vi "13-2 시리얼통신.vi"() -> ()   [LabVIEW 2014]
uses:
  <vilib>/Instr/_visa.llb/VISA Configure Serial Port (Instr).vi
panel:
  in  "설정":bool
  in  "TH500 통신":bool
  in  "정지":bool
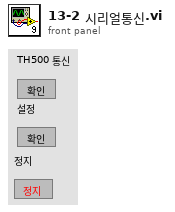
[diagram p1: front panel]
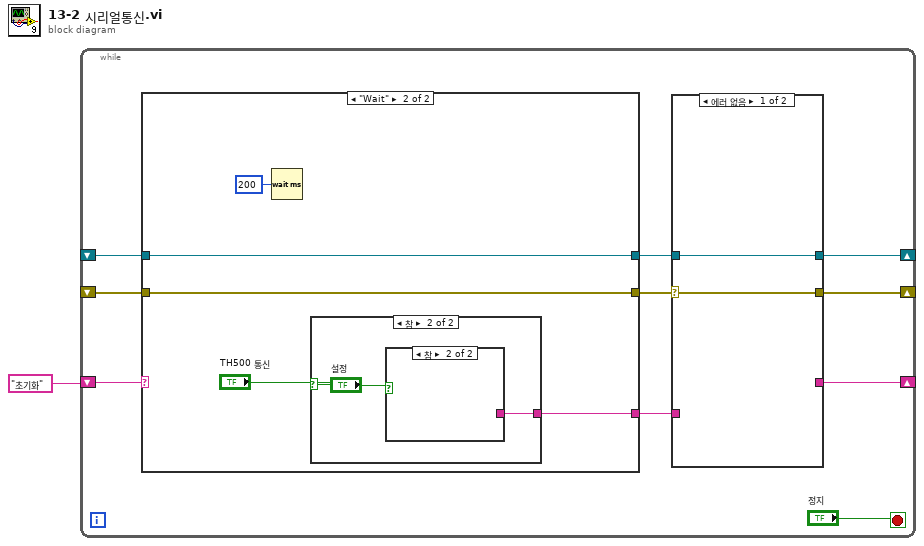
[diagram p0: block diagram]
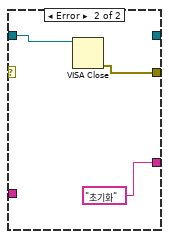
[diagram p2: hidden frame]
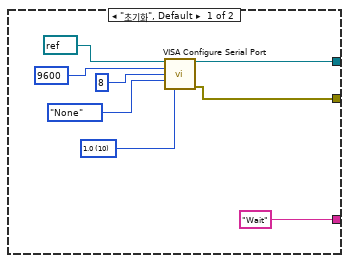
[diagram p3: hidden frame]
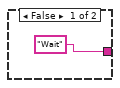
[diagram p4: hidden frame]
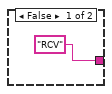
[diagram p5: hidden frame]
diagram:
  n1 = while {
    shift-right: [w6] -> _
    shift-left: _ -> [w2]
    shift-right: [w5] -> _
    shift-left: _ -> [w3]
    shift-right: [w4] -> _
    shift-left: "초기화" -> [w11]
    stop <- "정지" stop-if-true
    n2 = case shown="\"Wait\"" w11 {
      tunnel: ["Wait" w26] -> w9
      tunnel: [w18 w29] -> w8
      tunnel: [w17 w28] -> w7
      tunnel: w3 -> [_ w29]
      tunnel: w2 -> [_ w28]
      frame "초기화", Default {
        w20 = u16 10 items=["1.0"=10, "1.5"=15, "2.0"=20] ("stop bits (10: 1 bit)")
        n3 = call-poly "VISA Configure Serial Port"("VISA resource name"=refnum<visa-resource-name> refnum, "baud rate (9600)"=u32 9600, "data bits (8)"=u16 8, "parity (0:none)"=enum16{"None", "Odd", "Even", "Mark", "Space"}."None", "stop bits (10: 1 bit)"=w20) -> ("VISA resource name out"=w17:refnum<visa-resource-name>, "error out"=w18:errorcluster)  [unwired: 9 in]
      }
      frame "Wait" {
        n4 = Wait (ms)(milliseconds to wait=u32 200 ("대기 시간(ms)")) -> ()  [unwired: 1 out]
        n5 = case shown="참" "TH500 통신" {
          tunnel: ["Wait" w31] -> w26
          frame False {
          }
          frame True {
            n6 = case shown="참" "설정" {
              tunnel: ["RCV" _] -> w31
              frame False {
              }
              frame True {
              }
            }
          }
        }
      }
    }
    n7 = case shown="에러 없음" w8 {
      selector: w8 -> [w12 _]
      tunnel: w9 -> [_ _]
      tunnel: w7 -> [w13 w16]
      tunnel: [w13 _] -> w6
      tunnel: [w12 w15] -> w5
      tunnel: [_ "초기화"] -> w4
      frame No Error {
      }
      frame Error {
        n8 = VISA Close(VISA resource name=w16) -> (error out=w15:errorcluster)  [unwired: 1 in]
      }
    }
  }
